vi "Dynamic call-Error message window.vi"(8 "error in (no error)":errorcluster, 11 "Error Message":string) -> (0 "error out":errorcluster)   [LabVIEW 2020]
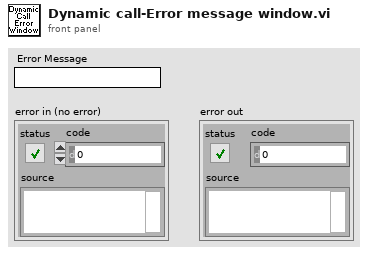
[diagram p1: front panel]
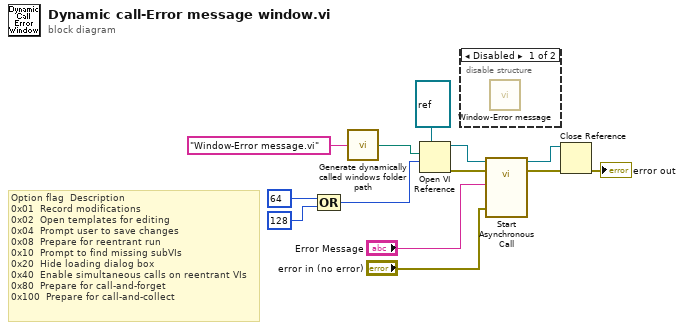
[diagram p0: block diagram]
diagram:
  # "Option flag \tDescription\n0x01 \tRecord modifications\n0x02 \tOpen templates for editing\n0x04 \tPrompt user to save changes\n0x08 \tPrepare for reentrant run\n0x10 \tPrompt to find missing subVIs\n0x20 \tHide loading dialog box\n0x40 \tEnable simultaneous calls on reentrant VIs\n0x80 \tPrepare for call-and-forget\n0x100 \tPrepare for call-and-collect"
  n1 = Compound Arithmetic op=OR(64, 128) -> (w7:i32)
  n2 = call "Generate dynamically called windows folder path.vi"("name of dynamically called VI"="Window-Error message.vi" ("Error Source")) -> ("Dynamically called VI path"=w11:path)
  n3 = Open VI Reference(type specifier VI Refnum (for type only)=refnum<vi> refnum, vi path=w11, options=w7) -> (vi reference=w8:refnum<vi>, error out=w9:errorcluster)  [unwired: 3 in]
  n4 = disable-structure shown="Disabled" {
    frame Disabled {
      n5 = call "Window-Error message.vi"() -> ()  [unwired: 11 in, 1 out]
    }
    frame Enabled {
    }
  }
  n6 = call-by-ref "Start Asynchronous Call"(reference=w8, error in=w9, 8:"error in (no error)"="error in (no error)", "Message"="Error Message") -> (reference out=w2:refnum<vi>, error out=w3:errorcluster)  [unwired: 9 in, 1 out]
  n7 = Close Reference(reference=w2, error in (no error)=w3) -> (error out=→"error out":errorcluster)
